vi "Subtract (Elementwise) - C,CM.vi"(1 "Complex Matrix A":T1, 2 "Complex Scalar c":cdb) -> (0 "c - A":T1)   [LabVIEW 2010, in "NI_Matrix.lvlib"]
doc: "Computes the difference of the inputs."
uses:
  NI_Matrix.lvlib
  ComplexMatrix.ctl
  Matrix To Array - CM.vi
  Array To Matrix - CA2.vi
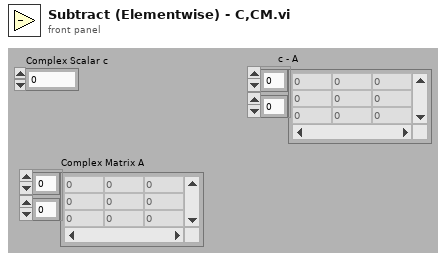
[diagram p1: front panel]
types:
  T1 = typedef "NI_Matrix.lvlib/ComplexMatrix.ctl" = cdb[][]
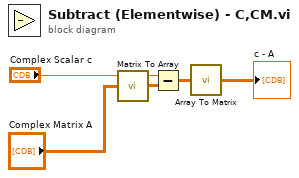
[diagram p0: block diagram]
diagram:
  n1 = call-poly "Matrix To Array.vi"("Complex Matrix"="Complex Matrix A") -> ("Complex 2D Array"=w2:cdb[][])
  n2 = Subtract(x="Complex Scalar c", y=w2) -> (x-y=w4:cdb[][])
  n3 = call-poly "Array To Matrix.vi"("Complex 2D Array"=w4) -> ("Complex Matrix"=→"c - A":T1)
